vi "LVDimInterface.dim_get_service_info.vi"(0 "callBackID":i32, 5 "error in (no error)":errorcluster) -> (10 "quality":i32, 11 "refNum":u32, 12 "timeStamp":dbl, 13 "serviceID":u32, 14 "callBackID (out)":i32, 15 "serviceName":string, 16 "typeDescriptor":string, 17 "callBackType":i32, 18 "refNumType":i32, 19 "error out":errorcluster)   [LabVIEW 2013, in "LVDimInterface.lvlib"]
doc: "Gets information about a DIM (command) service to which a callback is registered.\n\nThis VI can be used to get information about a DIM command (= to be used by a DIM server) or to get information about a DIM service (= to be used by a client). \n\nHistory: 13-FEB-2006, Dietrich Beck\n\nCopyright (C)\nGesellschaft für Schwerionenforschung, GSI\nPlanckstr. 1\n64291 Darmstadt\nGermany\n\nContact: D.Beck@gsi.de \n\nThis program is free software; you can redistribute it and/or modify it under the terms of the \nGNU General Public License as published by the Free Software Foundation; either version 2 of the license, or (at your option) any later version.\n\nThis program is distributed in the hope that it will be useful, but WITHOUT ANY WARRANTY; without even the implied warranty of MERCHANTABILITY or FITNESS FOR A PARTICULAR PURPOSE. See the GNU General License for more details (http://www.gnu.org).\n\nGesellschaft für Schwerionenforschung, GSI\nPlanckstr. 1, 64291 Darmstadt, Germany\nFor all questions and ideas contact D. Beck.\nLast update: 16-DEC-2005"
uses:
  LVDimInterface.lvlib
  bin/libDimWrapper.dll
  C/GPL/Projects/DimLVEvent/bin/libDimWrapper.so
  C/GPL/Projects/DimLVEvent/bin/libDimWrapperSPL.dll
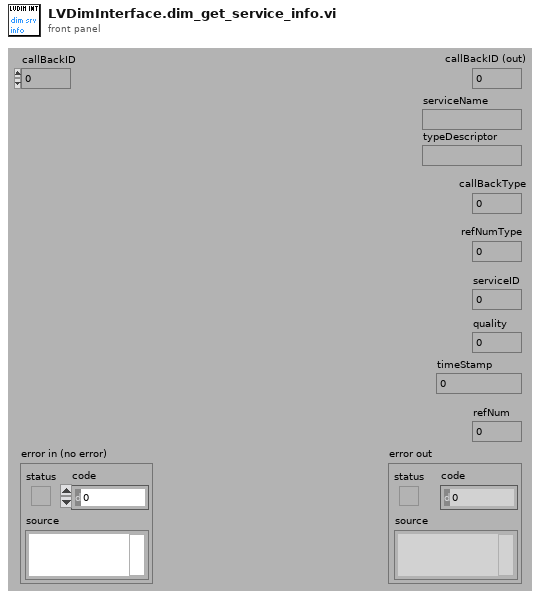
[diagram p1: front panel]
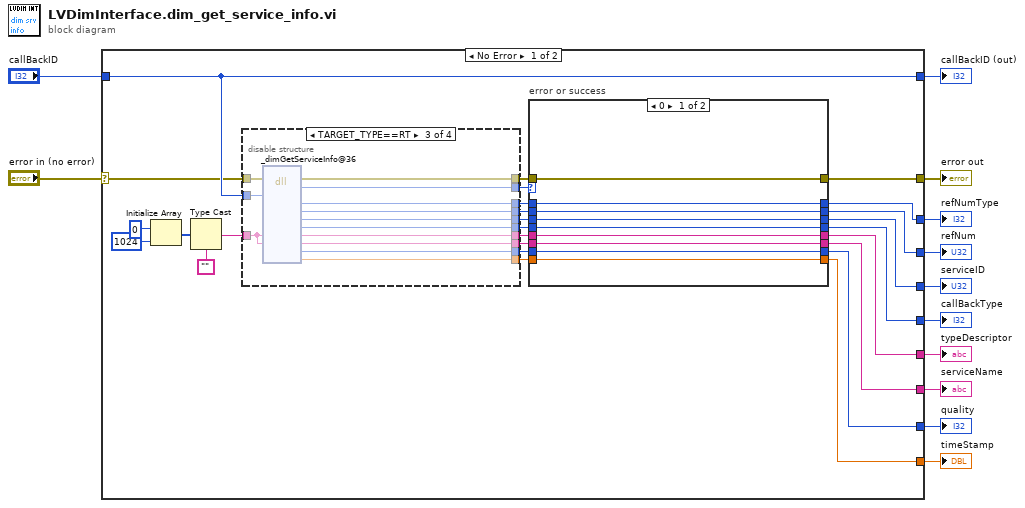
[diagram p0: block diagram]
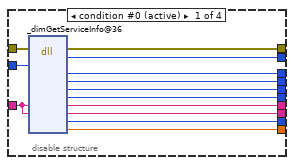
[diagram p2: hidden frame]
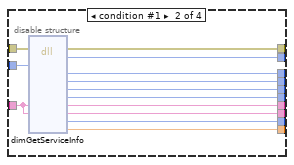
[diagram p3: hidden frame]
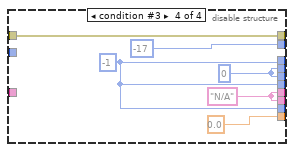
[diagram p4: hidden frame]
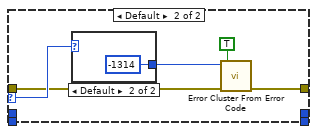
[diagram p5: hidden frame]
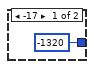
[diagram p6: hidden frame]
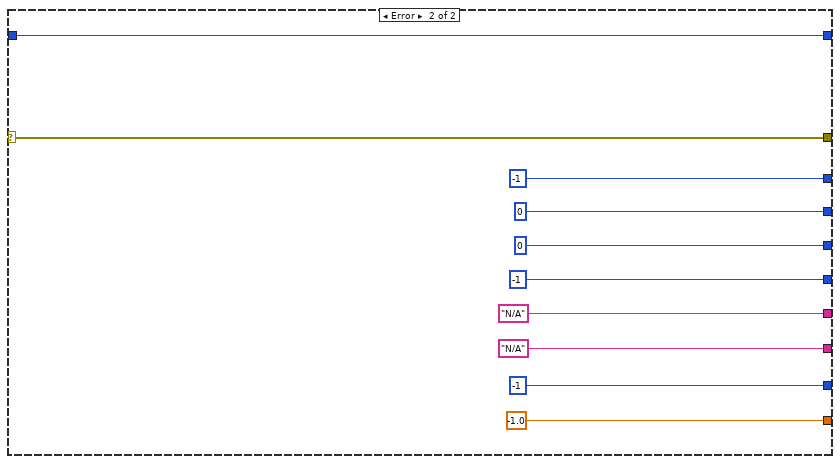
[diagram p7: hidden frame]
diagram:
  n1 = case shown="No Error" "error in (no error)" {
    selector: "error in (no error)" -> [w14 w104]
    tunnel: "callBackID" -> [w36 w109]
    tunnel: [w29 -1 ("refNumType")] -> w11
    tunnel: [w25 u32 0 ("serviceID")] -> w10
    tunnel: [w23 -1 ("callBackType")] -> w9
    tunnel: [w21 "N/A" ("typeDescriptor")] -> w8
    tunnel: [w37 w104] -> w7
    tunnel: [w36 w109] -> w5
    tunnel: [w19 "N/A" ("serviceName")] -> w4
    tunnel: [w17 -1 ("quality")] -> w3
    tunnel: [w15 -1.0 ("timeStamp")] -> w2
    tunnel: [w27 0 ("refNum")] -> w1
    frame No Error {
      n2 = Initialize Array(i8 0, 1024 ("dimension size")) -> (w33:i8[])
      n3 = Type Cast(type="" ("Empty String Constant"), x=w33) -> (*(type *) &x=w31:string)
      n4 = disable-structure "Conditional Disable Structure" shown="TARGET_TYPE==RT" {
        disable-tunnel: [w51 w64 w77 -17 ("error")] -> w38
        disable-tunnel: w36 -> [w50 w63 w76 _]
        disable-tunnel: w31 -> [w49 w62 w75 _]
        disable-tunnel: [w48 w61 w74 w80] -> w30
        disable-tunnel: [w47 w60 w73 w82] -> w28
        disable-tunnel: [w46 w59 w72 w82] -> w26
        disable-tunnel: [w45 w58 w71 w80] -> w24
        disable-tunnel: [w44 w57 w70 w81] -> w22
        disable-tunnel: [w43 w56 w69 w81] -> w20
        disable-tunnel: [w42 w55 w68 w80] -> w18
        disable-tunnel: [w41 w54 w67 0.0 ("timeStamp")] -> w16
        disable-tunnel: w14 -> [w39 w52 w66 w78]
        disable-tunnel: [w40 w53 w65 w78] -> w13
        frame condition #0 (active) {
          n5 = dll-call lib="C:/User/Brand/LVP/Submodules/DimLVEvent/bin/libDimWrapper.dll" fn="_dimGetServiceInfo@36"(error in=w39, "callBackID"=w50, "typeDesc"=w49, "serviceName"=w49) -> (error out=w40:errorcluster, "error"=w51:i32, "refNumType"=w48:i32, "refNum"=w47:u32, "serviceID"=w46:u32, "callBackType"=w45:i32, "typeDesc"=w44:string, "serviceName"=w43:string, "quality"=w42:i32, "timeStamp"=w41:dbl)  [unwired: 9 in, 1 out]
        }
        frame condition #1 {
          n6 = dll-call lib="F:/LVSCC/C/GPL/Projects/DimLVEvent/bin/libDimWrapper.so" fn="dimGetServiceInfo" label="libDimWrapper.dll:_dimGetServiceInfo@36"(error in=w52, "callBackID"=w63, "typeDesc"=w62, "serviceName"=w62) -> (error out=w53:errorcluster, "error"=w64:i32, "refNumType"=w61:i32, "refNum"=w60:u32, "serviceID"=w59:u32, "callBackType"=w58:i32, "typeDesc"=w57:string, "serviceName"=w56:string, "quality"=w55:i32, "timeStamp"=w54:dbl)  [unwired: 9 in, 1 out]
        }
        frame condition #2 {
          n7 = dll-call lib="C:/User/Brand/SVN/C/GPL/Projects/DimLVEvent/bin/libDimWrapperSPL.dll" fn="_dimGetServiceInfo@36"(error in=w66, "callBackID"=w76, "typeDesc"=w75, "serviceName"=w75) -> (error out=w65:errorcluster, "error"=w77:i32, "refNumType"=w74:i32, "refNum"=w73:u32, "serviceID"=w72:u32, "callBackType"=w71:i32, "typeDesc"=w70:string, "serviceName"=w69:string, "quality"=w68:i32, "timeStamp"=w67:dbl)  [unwired: 9 in, 1 out]
        }
        frame condition #3 {
          w81 = "N/A" ("typeDesc")
          w82 = u32 0 ("refNum")
          w80 = -1 ("refNumType")
        }
      }
      n8 = case "error or success" shown="0" w38 {
        selector: w38 -> [_ w97]
        tunnel: [w84 w96] -> w37
        tunnel: [w92 _] -> w29
        tunnel: w30 -> [w92 _]
        tunnel: [w91 _] -> w27
        tunnel: w28 -> [w91 _]
        tunnel: [w90 _] -> w25
        tunnel: w26 -> [w90 _]
        tunnel: [w89 _] -> w23
        tunnel: w24 -> [w89 _]
        tunnel: [w88 _] -> w21
        tunnel: w22 -> [w88 _]
        tunnel: [w87 _] -> w19
        tunnel: w20 -> [w87 _]
        tunnel: [w86 _] -> w17
        tunnel: w18 -> [w86 _]
        tunnel: [w85 _] -> w15
        tunnel: w16 -> [w85 _]
        tunnel: w13 -> [w84 w93]
        frame 0 {
        }
        frame Default {
          n9 = case shown="Default" w97 {
            tunnel: [-1320 ("code") -1314 ("code")] -> w94
            frame -17 {
            }
            frame Default {
            }
          }
          n10 = call <vilib>:"Error Cluster From Error Code.vi"("show call chain? (False)"=TRUE ("status"), "error in (no error)"=w93, "error code (0)"=w94) -> ("error out"=w96:errorcluster)  [unwired: 6 in]
        }
      }
    }
    frame Error {
    }
  }
  "error out" <- w7
  "callBackID (out)" <- w5
  "typeDescriptor" <- w8
  "refNumType" <- w11
  "serviceID" <- w10
  "callBackType" <- w9
  "serviceName" <- w4
  "quality" <- w3
  "timeStamp" <- w2
  "refNum" <- w1
